vi "Write Config File.vi"(8 "error in (no error)":errorcluster, 10 "Config File":path, 11 "Node Ptr":T1 format="%.0x") -> (0 "error out":errorcluster, 3 "Node Ptr out":T1 format="%.0x")   [LabVIEW 2019, in "UDP-Custom-Device System Explorer.lvlib" / "Shared Channel Accessors.lvlib"]
uses:
  Shared Channel Accessors.lvlib
  <vilib>/NI VeriStand/Custom Device API/Custom Device Item Ref.ctl
  Shared/Constants.vi
  <vilib>/NI VeriStand/Custom Device API/Set Item Property (Path).vi
  <vilib>/NI VeriStand/Custom Device API/Custom Device API.lvlib
  Shared/UDP-Custom-Device Shared.lvlib
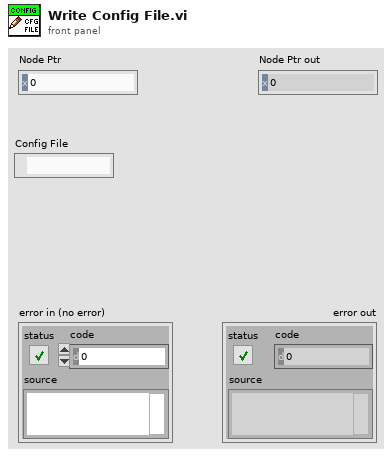
[diagram p1: front panel]
types:
  T1 = typedef "Custom Device API.lvlib/Custom Device Item Ref.ctl" = u64
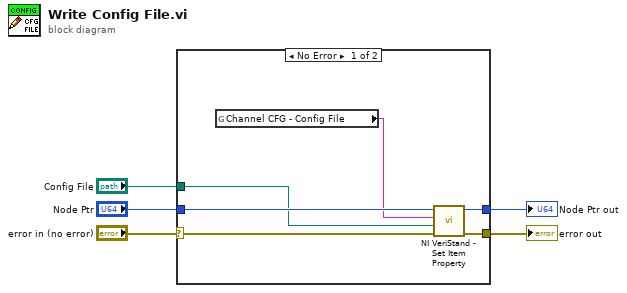
[diagram p0: block diagram]
diagram:
  n1 = case shown="No Error" "error in (no error)" {
    selector: "error in (no error)" -> [w6 w12]
    tunnel: [w11 w12] -> w5
    tunnel: "Node Ptr" -> [w10 w13]
    tunnel: [w9 w13] -> w3
    tunnel: "Config File" -> [w8 _]
    frame No Error {
      n2 = global read "Constants.vi" "Channel CFG - Config File"() -> (w7:string)
      n3 = call-poly <vilib>:"NI VeriStand - Set Item Property.vi"("error in (no error)"=w6, "Value"=w8, "Property Name"=w7, "Item Ref in"=w10) -> ("error out"=w11:errorcluster, "Item Ref out"=w9:T1)  [unwired: 5 in, 1 out]
    }
    frame Error {
    }
  }
  "error out" <- w5
  "Node Ptr out" <- w3
